vi "Configure Test Branching.vi"(8 "error in (no error)":errorcluster, 9 "Destination Block (1)":u32=1, 10 "Program Behavior (0: Jump on Pass)":u16(ring) items=["Jump on Pass", "Jump on Failure", "Don't Jump"], 11 "VISA resource name":refnum<visa-resource-name>) -> (0 "error out":errorcluster, 3 "VISA resource name out":refnum<visa-resource-name>)   [LabVIEW 2015, in "Keithley 24XX.lvlib"]
doc: "Configure the next memory destination based on the results of this memory block's tests."
uses:
  <instrlib>/Keithley 24XX/Keithley 24XX.lvlib
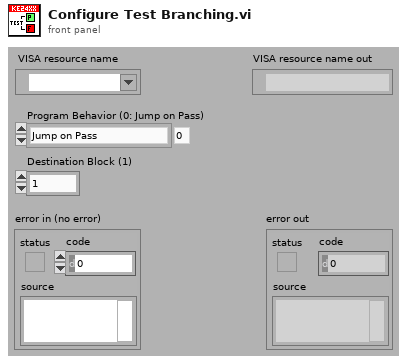
[diagram p1: front panel]
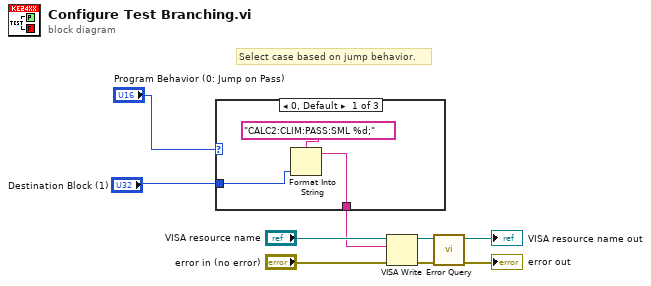
[diagram p0: block diagram]
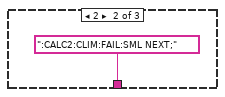
[diagram p2: hidden frame]
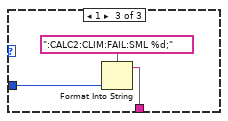
[diagram p3: hidden frame]
diagram:
  # "Select case based on jump behavior."
  n1 = case shown="0, Default" "Program Behavior (0: Jump on Pass)" {
    tunnel: "Destination Block (1)" -> [w10 _ w16]
    tunnel: [w11 ":CALC2:CLIM:FAIL:SML NEXT;" w14] -> w2
    frame 0, Default {
      n2 = Format Into String(format string="CALC2:CLIM:PASS:SML %d;", w10) -> (resulting string=w11:string)  [unwired: 2 in, 1 out]
    }
    frame 2 {
    }
    frame 1 {
      n3 = Format Into String(format string=":CALC2:CLIM:FAIL:SML %d;", w16) -> (resulting string=w14:string)  [unwired: 2 in, 1 out]
    }
  }
  n4 = VISA Write(VISA resource name="VISA resource name", write buffer=w2, error in (no error)="error in (no error)") -> (VISA resource name out=w5:refnum<visa-resource-name>, error out=w4:errorcluster)  [unwired: 1 out]
  n5 = call <instrlib>:"Error Query.vi"("error in (no error)"=w4, "VISA resource name"=w5) -> ("error out"=→"error out":errorcluster, "VISA resource name out"=→"VISA resource name out":refnum<visa-resource-name>)  [unwired: 6 in, 2 out]
